vi "Create.vi"(8 "Error In":errorcluster, 11 "Reader":refnum<class "Abstract.lvclass">) -> (0 "Error Out":errorcluster, 3 "Render":refnum<class "Render.lvclass">)   [LabVIEW 2018, in "Toolkit.lvlib" / "Render.lvclass"]
uses:
  Render.lvclass
  Readers/Abstract/Abstract.lvclass
  Render.lvclass/Render.ctl
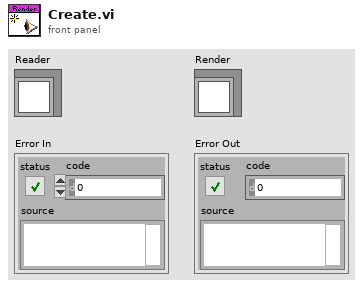
[diagram p1: front panel]
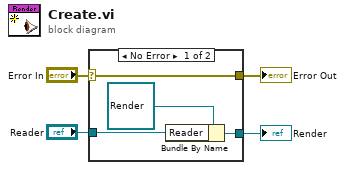
[diagram p0: block diagram]
diagram:
  n1 = case shown="No Error" "Error In" {
    selector: "Error In" -> [w6 w9]
    tunnel: [w6 w9] -> w3
    tunnel: "Reader" -> [w7 _]
    tunnel: [w5 _] -> w1
    frame No Error {
      n2 = Bundle By Name(cluster=refnum<class "Render.lvclass"> refnum ("Toolkit.lvlib:Render.lvclass"), "Reader"=w7) -> (w5:refnum<class "Render.lvclass">)
    }
    frame Error {
    }
  }
  "Error Out" <- w3
  "Render" <- w1
